vi "Array of Clusters to Map.vi"(8 "error in":errorcluster, 11 "Array of Clusters (key-value)":variant) -> (0 "error out":errorcluster, 3 "Map":variant)   [LabVIEW 2020, in "JSONtext.lvlib" / "SetMap.lvlib"]
uses:
  <vilib>/JDP Science/JSONtext/support/Set Map/SetMap.lvlib
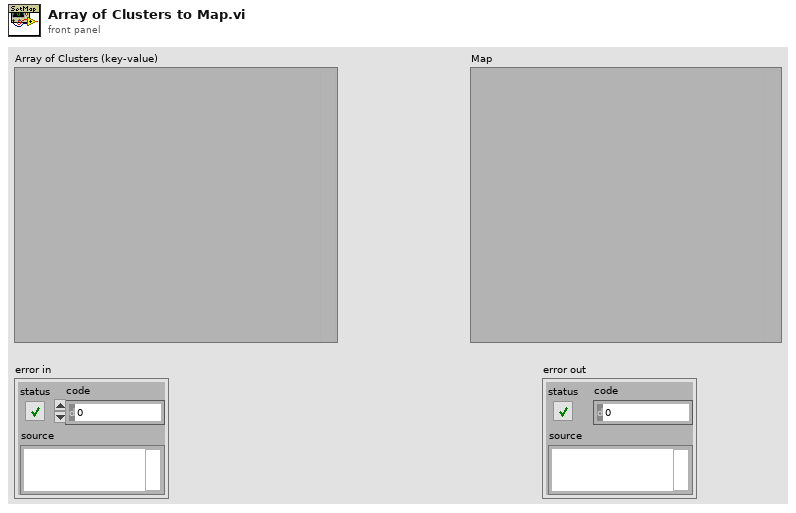
[diagram p1: front panel]
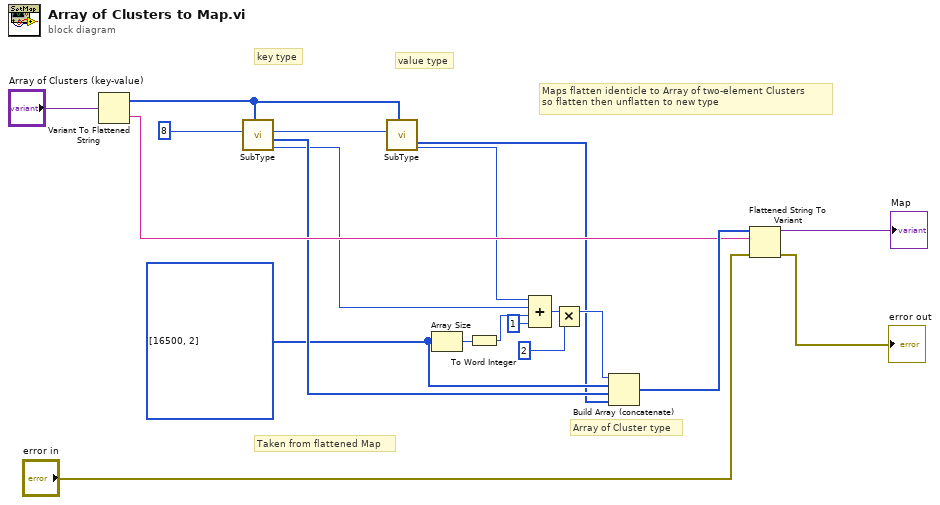
[diagram p0: block diagram]
diagram:
  w11 = i16[] [16500, 2] ("type string 7")
  # "Taken from flattened Map"
  # "Maps flatten identicle to Array of two-element Clusters\nso flatten then unflatten to new type"
  # "value type"
  # "key type"
  # "Array of Cluster type"
  n1 = Variant To Flattened String(Variant="Array of Clusters (key-value)") -> (data string=w13:string, 1:w1:i16[])
  n2 = call <vilib>:"SubType.vi"("type"=w1, "Offset In"=i16 8 ("index")) -> ("Size"=w5:i16, "subtype"=w12:i16[], "Offset out"=w4:i16)  [unwired: 7 in]
  n3 = call <vilib>:"SubType.vi"("type"=w1, "Offset In"=w4) -> ("Size"=w2:i16, "subtype"=w3:i16[])  [unwired: 7 in, 1 out]
  n4 = Array Size(array=w11) -> (size(s)=w10:i32)
  n5 = To Word Integer(number=w10) -> (16bit integer=w8:i16)
  n6 = Compound Arithmetic op=ADD(w2, w5, w8, i16 1 ("value")) -> (w9:i16)
  n7 = Multiply(x=w9, y=i16 2) -> (x*y=w15:i16)
  n8 = Build Array (concatenate)(w15, w11, w12, w3) -> (w14:i16[])
  n9 = Flattened String To Variant(4:"error in", 6:w13, 7:w14) -> (0:→"error out":errorcluster, 3:→"Map":variant)
